vi "queue.vi"() -> ()   [LabVIEW 2018]
panel:
  out "element 2":bool
  out "element":bool
  in  "OK Button":bool
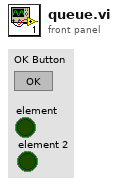
[diagram p1: front panel]
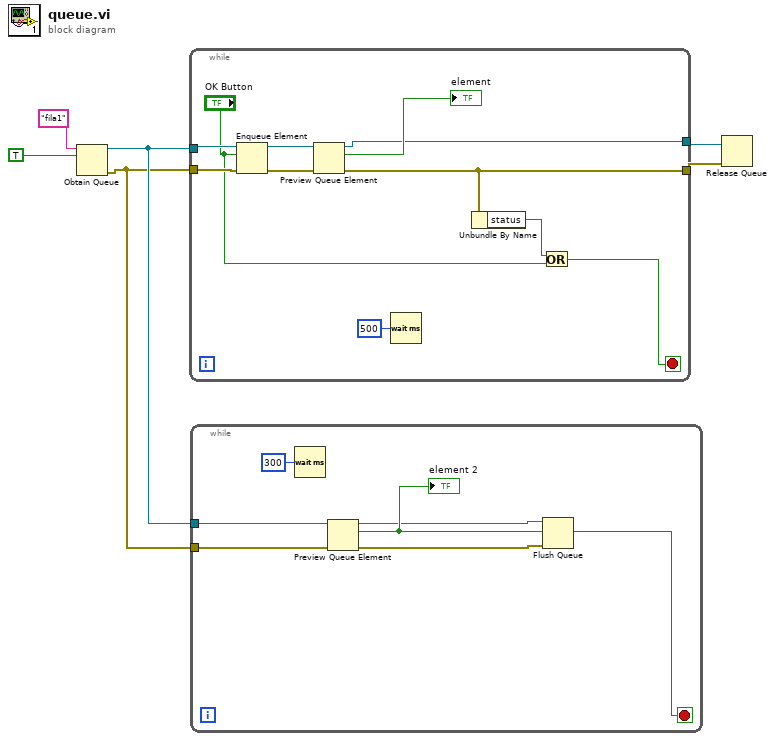
[diagram p0: block diagram]
diagram:
  n1 = Obtain Queue(name (unnamed)="fila1", element data type=TRUE) -> (queue out=w2:refnum<queue>, error out=w1:errorcluster)  [unwired: 3 in, 1 out]
  n2 = while {
    tunnel: w2 -> [w17]
    tunnel: w1 -> [w16]
    tunnel: [w12] -> w4
    tunnel: [w11] -> w3
    stop <- w8 stop-if-true
    n3 = Enqueue Element(queue=w17, element="OK Button", error in (no error)=w16) -> (queue out=w15:refnum<queue>, error out=w14:errorcluster)  [unwired: 1 in, 1 out]
    n4 = Preview Queue Element(queue=w15, error in (no error)=w14) -> (queue out=w12:refnum<queue>, element=→"element":bool, error out=w11:errorcluster)  [unwired: 1 in, 1 out]
    n5 = Wait (ms)(milliseconds to wait=u32 500) -> ()  [unwired: 1 out]
    n6 = Unbundle By Name(w11) -> ("status"=w10:bool)
    n7 = Or(x=w10, y="OK Button") -> (x .or. y?=w8:bool)
  }
  n8 = while {
    tunnel: w2 -> [w23]
    tunnel: w1 -> [w22]
    stop <- w21 stop-if-true
    n9 = Wait (ms)(milliseconds to wait=u32 300) -> ()  [unwired: 1 out]
    n10 = Preview Queue Element(queue=w23, error in (no error)=w22) -> (queue out=w20:refnum<queue>, element=w21:bool, error out=w19:errorcluster)  [unwired: 1 in, 1 out]
    "element 2" <- w21
    n11 = Flush Queue(queue=w20, error in (no error)=w19) -> ()  [unwired: 3 out]
  }
  n12 = Release Queue(queue=w4, error in (no error)=w3) -> ()  [unwired: 1 in, 3 out]
